vi "SNRvariations.vi"() -> ()   [LabVIEW 2012]
uses:
  <vilib>/addons/Modulation/Digital/General/MT Generate PSK System Parameters(M).vi
  <instrlib>/niUSRP/niUSRP Write Tx Data (CDB Cluster).vi
  <vilib>/addons/Modulation/niDMT.lvlib
panel:
  out "coerced gain":dbl format="%#_6f"
  out "coerced carrier frequency":dbl=100000.0 format="%#_6p"
  in  "IQ rate":dbl=100000.0 format="%#_6p"
  in  "active antenna":string
  in  "Carrier Frequency":dbl
  out "x+y":dbl
  out "Tx Frequency [Hz]":dbl
  out "Enter control signal (1,2 or 3) 2":string
  out "String":string
  in  "millisecond multiple":u32
  out "millisecond timer value":u32
  out "Message Text 2":string
  out "Symbol Rate\n[symbols/sec]":dbl=25000.0 format="%#.6p"
  in  "BPSK System Parameters 9":T1={"Samples per Symbol"=8, "symbol map"=[], "Differential PSK"=enum."disable", "PSK type"=0} caption="BPSK System Parameters" {"PSK type" items=["normal", "shifted", "offset"]; "symbol map" format="%.3f"}
  in  "BPSK System Parameters 8":T1={"Samples per Symbol"=8, "symbol map"=[], "Differential PSK"=enum."disable", "PSK type"=0} caption="BPSK System Parameters" {"PSK type" items=["normal", "shifted", "offset"]; "symbol map" format="%.3f"}
  in  "BPSK System Parameters 7":T1={"Samples per Symbol"=8, "symbol map"=[], "Differential PSK"=enum."disable", "PSK type"=0} caption="BPSK System Parameters" {"PSK type" items=["normal", "shifted", "offset"]; "symbol map" format="%.3f"}
  in  "BPSK System Parameters 6":T1={"Samples per Symbol"=8, "symbol map"=[], "Differential PSK"=enum."disable", "PSK type"=0} caption="BPSK System Parameters" {"PSK type" items=["normal", "shifted", "offset"]; "symbol map" format="%.3f"}
  in  "BPSK System Parameters 5":T1={"Samples per Symbol"=8, "symbol map"=[], "Differential PSK"=enum."disable", "PSK type"=0} caption="BPSK System Parameters" {"PSK type" items=["normal", "shifted", "offset"]; "symbol map" format="%.3f"}
  in  "BPSK System Parameters 4":T1={"Samples per Symbol"=8, "symbol map"=[], "Differential PSK"=enum."disable", "PSK type"=0} caption="BPSK System Parameters" {"PSK type" items=["normal", "shifted", "offset"]; "symbol map" format="%.3f"}
  in  "BPSK System Parameters 3":T1={"Samples per Symbol"=8, "symbol map"=[], "Differential PSK"=enum."disable", "PSK type"=0} caption="BPSK System Parameters" {"PSK type" items=["normal", "shifted", "offset"]; "symbol map" format="%.3f"}
  in  "Tab Control":T2(tab)
  in  "Enter control signal (1,2 or 3)":string
  in  "Packet Parameters":T3={"Guard Bits "=30, "Sync Bits"=20, "Message Bits"=128}
  in  "Packet Pad \n[samples]":i32=200
  in  "Blank Frame \n[samples]":i32=500
  out "Number of Packets in Message":i32=46
  in  "PN sequence order\nfor Sync Bits":i32=31 caption="PN sequence order (9)"
  in  "Packet Repeat":i32=2
  in  "Pulse Shaping Filter Parameters":T4={"Alpha"=0.5, "Filter Length"=6, "TX Filter"=enum."Root Raised Cos"} caption="Pulse Shaping Filter" {"Alpha" format="%.2f"}
  in  "USRP IP address":refnum<k15>="192.168.10.2"
  out "error out":errorcluster
  in  "Queue Length":i32=10
  in  "stop":bool
  out "result":bool
  out "Constellation Graph":T5(graph)
  in  "autoscale":bool
  in  "millisecond multiple 2":u32
  out "millisecond timer value 2":u32
  out "x = y?":bool
  out "Boolean":bool
  out "M-PSK (4)":i32
  # "Guard\nBand"
  # "Sync\nSeq"
  # "Packet\nNumber"
  # "Pad\nData"
  # "Blank\nFrame"
  # "Data"
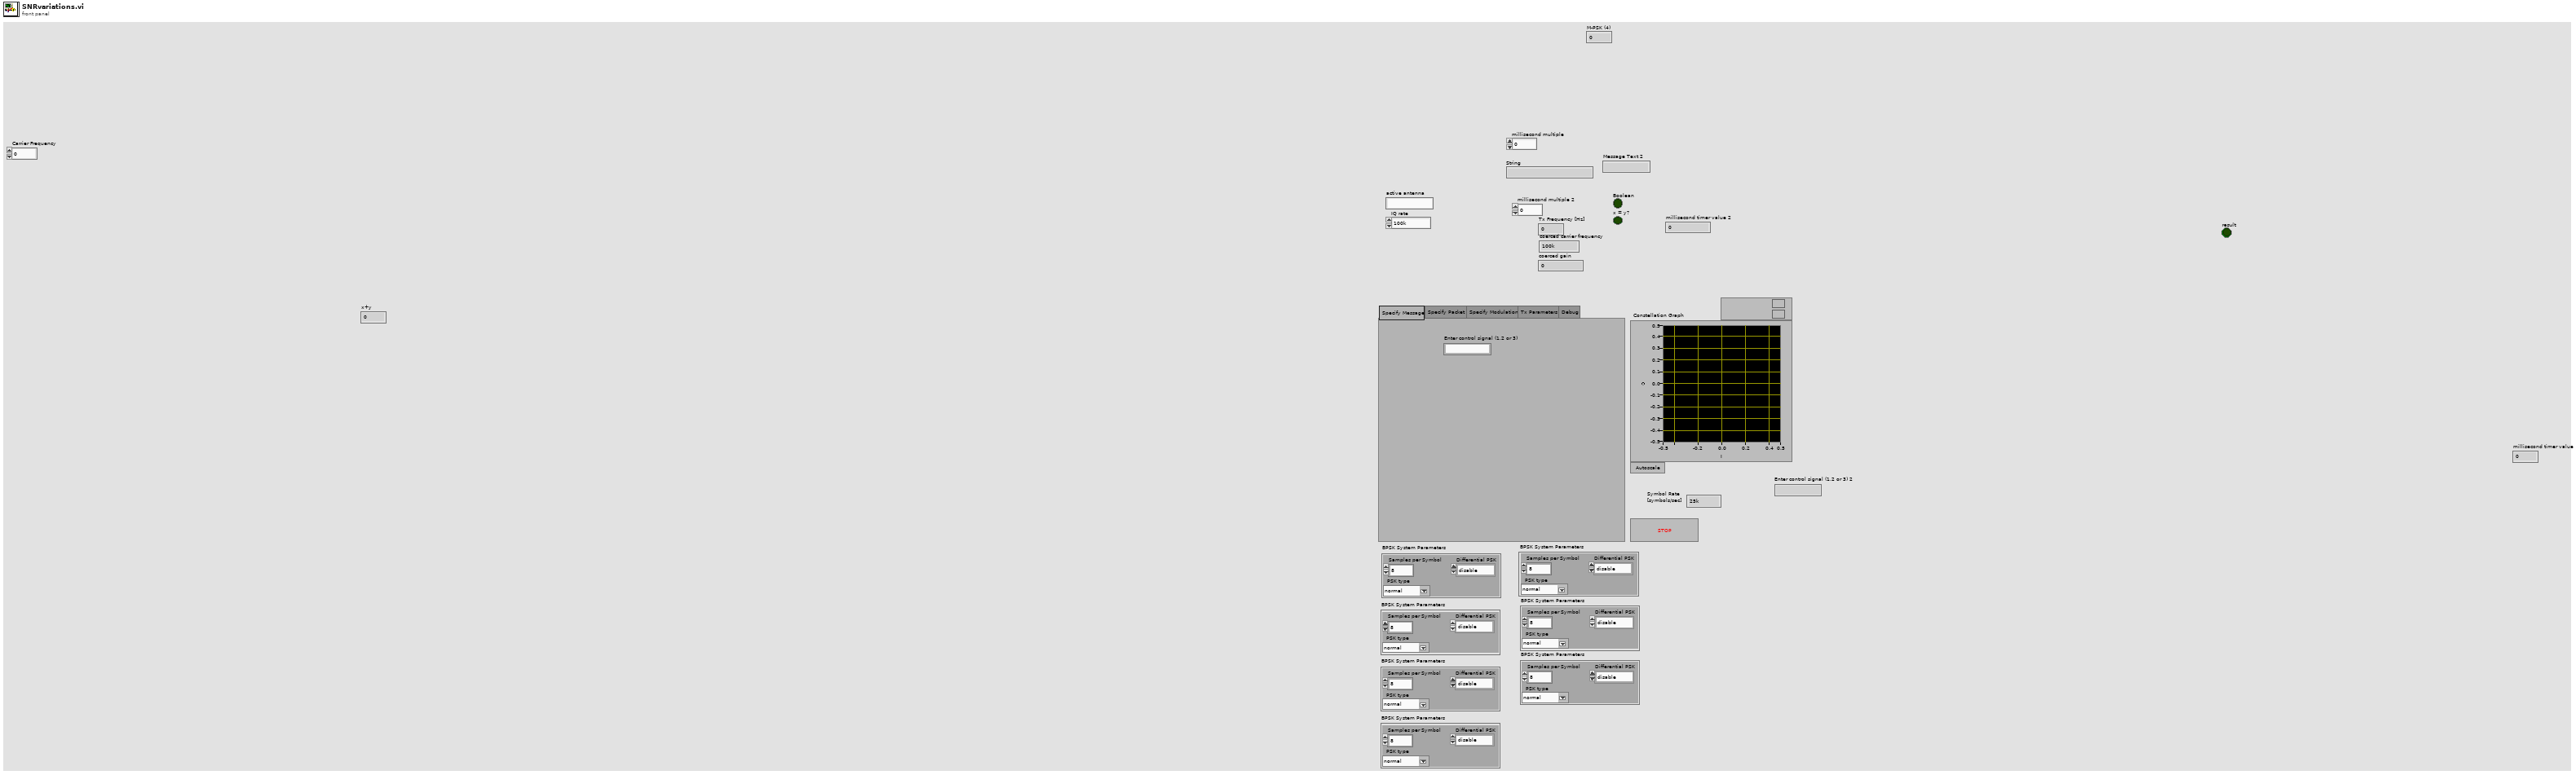
[diagram p1: front panel]
types:
  T1 = cluster{"Samples per Symbol":i32, "symbol map":cdb[], "Differential PSK":enum16{"disable", "enable"}, "PSK type":u16}
  T2 = enum32{"Specify Message", "Specify Packet", "Specify Modulation", "Tx Parameters", "Debug"}
  T3 = cluster{"Guard Bits ":i32, "Sync Bits":i32, "Message Bits":i32}
  T4 = cluster{"Alpha":dbl, "Filter Length":i32, "TX Filter":enum16{"none", "Raised Cosine", "Root Raised Cos", "Gaussian"}}
  T5 = cluster{"Decimated Array":dbl[], "Decimated Array":dbl[]}[]
  T6 = cluster{"samples per symbol (16)":i32, "symbol map":cdb[], "differential PSK":enum16{"disable", "enable"}, "PSK type":u16}
  T7 = cluster{"s? t:f":cluster{"t0":dbl, "dt":dbl, "Y":cdb[]}, i32}
  T8 = cluster{"output complex waveform":cluster{"t0":dbl, "dt":dbl, "Y":cdb[]}, i32}
  T9 = cluster{"constellation":dbl[], "oversampled data":dbl[]}[]
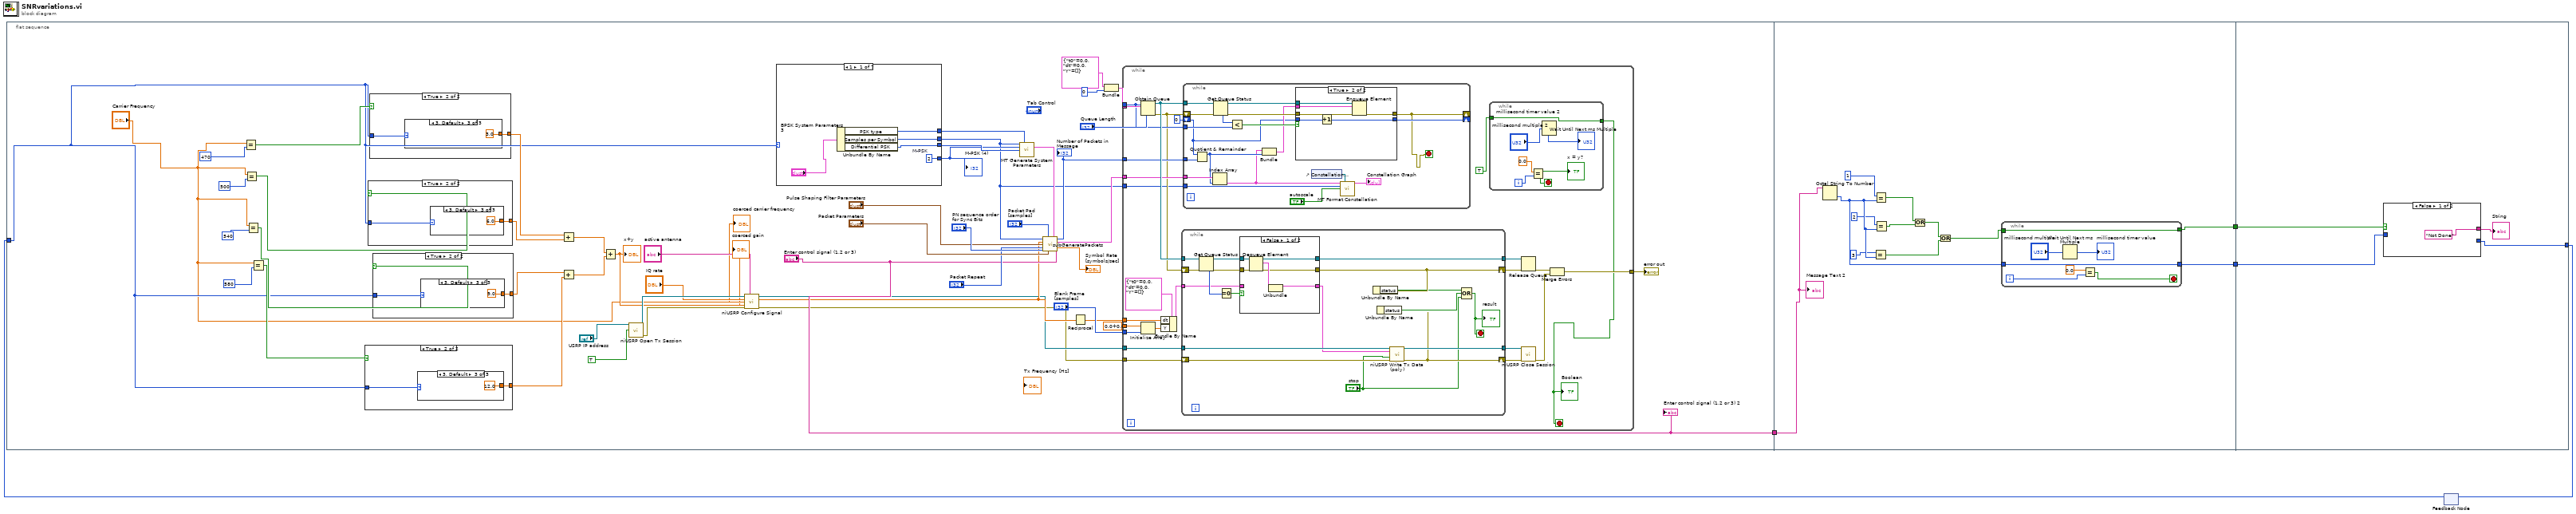
[diagram p0: block diagram]
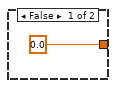
[diagram p2: hidden frame]
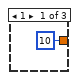
[diagram p3: hidden frame]
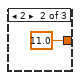
[diagram p4: hidden frame]
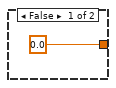
[diagram p5: hidden frame]
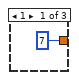
[diagram p6: hidden frame]
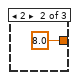
[diagram p7: hidden frame]
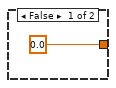
[diagram p8: hidden frame]
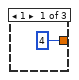
[diagram p9: hidden frame]
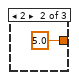
[diagram p10: hidden frame]
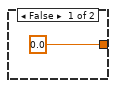
[diagram p11: hidden frame]
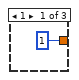
[diagram p12: hidden frame]
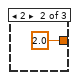
[diagram p13: hidden frame]
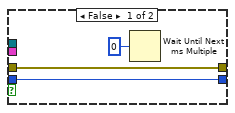
[diagram p14: hidden frame]
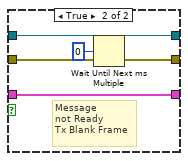
[diagram p15: hidden frame]
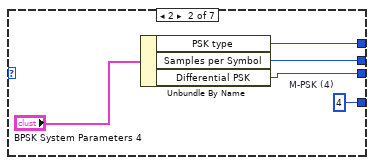
[diagram p16: hidden frame]
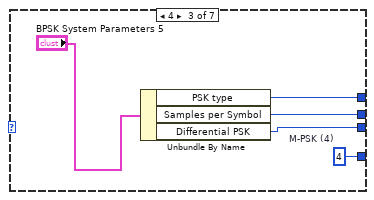
[diagram p17: hidden frame]
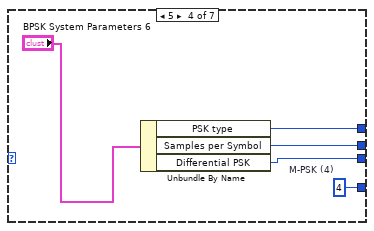
[diagram p18: hidden frame]
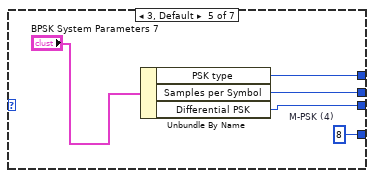
[diagram p19: hidden frame]
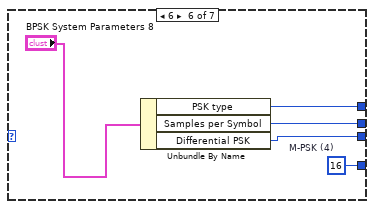
[diagram p20: hidden frame]
diagram:
  n1 = flat-sequence {
    tunnel: ["Enter control signal (1,2 or 3)"] -> w5
    tunnel: w1 -> [w13]
    tunnel: w5 -> [w202]
    tunnel: [w204] -> w4
    tunnel: [w203] -> w3
    tunnel: w4 -> [w223]
    tunnel: w3 -> [w222]
    tunnel: [w221] -> w2
    frame #0 {
      n2 = Equal?(x="Carrier Frequency", y=470) -> (x = y?=w14:bool)
      n3 = Equal?(x="Carrier Frequency", y=500) -> (x = y?=w15:bool)
      n4 = Equal?(x="Carrier Frequency", y=540) -> (x = y?=w16:bool)
      n5 = Equal?(x="Carrier Frequency", y=580) -> (x = y?=w17:bool)
      n6 = case shown="True" w17 {
        tunnel: [0.0 w57] -> w22
        tunnel: w13 -> [_ w58]
        frame False {
        }
        frame True {
          n7 = case shown="3, Default" w58 {
            tunnel: [10 11.0 12.0] -> w57
            frame 1 {
            }
            frame 2 {
            }
            frame 3, Default {
            }
          }
        }
      }
      n8 = case shown="True" w15 {
        tunnel: [0.0 w69] -> w24
        tunnel: w13 -> [_ w70]
        frame False {
        }
        frame True {
          n9 = case shown="3, Default" w70 {
            tunnel: [4 5.0 6.0] -> w69
            frame 1 {
            }
            frame 2 {
            }
            frame 3, Default {
            }
          }
        }
      }
      n10 = case shown="True" w14 {
        tunnel: [0.0 w75] -> w25
        tunnel: w13 -> [_ w76]
        frame False {
        }
        frame True {
          n11 = case shown="3, Default" w76 {
            tunnel: [1 2.0 3.0] -> w75
            frame 1 {
            }
            frame 2 {
            }
            frame 3, Default {
            }
          }
        }
      }
      n12 = case shown="True" w16 {
        tunnel: [0.0 w63] -> w23
        tunnel: w13 -> [_ w64]
        frame False {
        }
        frame True {
          n13 = case shown="3, Default" w64 {
            tunnel: [7 8.0 9.0] -> w63
            frame 1 {
            }
            frame 2 {
            }
            frame 3, Default {
            }
          }
        }
      }
      n14 = Add(x=w25, y=w24) -> (x+y=w27:dbl)
      n15 = Add(x=w23, y=w22) -> (x+y=w26:dbl)
      n16 = Add(x=w27, y=w26) -> (x+y=w12:dbl)
      "x+y" <- w12
      n17 = call <instrlib>:"niUSRP Open Tx Session.vi"("device names"="USRP IP address", "reset"=TRUE) -> ("session handle out"=w30:refnum<k15>, "error out"=w31:errorcluster)  [unwired: 12 in]
      n18 = call <instrlib>:"niUSRP Configure Signal.vi"("session handle"=w30, "IQ rate"="IQ rate", "carrier frequency"="Carrier Frequency", "gain"=w12, "error in (no error)"=w31, "active antenna"="active antenna") -> ("session handle out"=w29:refnum<k15>, "coerced IQ rate"=w32:dbl, "coerced carrier frequency"=→"coerced carrier frequency":dbl, "coerced gain"=→"coerced gain":dbl, "error out"=w28:errorcluster)  [unwired: 5 in]
      n19 = case shown="1" w13 {
        tunnel: [w168 w173 w180 w185 w190 w196 w199] -> w36
        tunnel: [w169 w174 w179 w184 w189 w195 w200] -> w55
        tunnel: [w171 w176 w181 w186 w188 w194 0 ("M-PSK (4)")] -> w47
        tunnel: [w170 w175 w178 w183 w191 w193 w201] -> w41
        frame 1 {
          w171 = 2  # M-PSK
          n20 = Unbundle By Name("BPSK System Parameters 3") -> ("PSK type"=w170:u16, "Samples per Symbol"=w168:i32, "Differential PSK"=w169:enum16{"disable", "enable"})
        }
        frame 2 {
          w176 = 4  # M-PSK (4)
          n21 = Unbundle By Name("BPSK System Parameters 4") -> ("PSK type"=w175:u16, "Samples per Symbol"=w173:i32, "Differential PSK"=w174:enum16{"disable", "enable"})
        }
        frame 4 {
          w181 = 4  # M-PSK (4)
          n22 = Unbundle By Name("BPSK System Parameters 5") -> ("PSK type"=w178:u16, "Samples per Symbol"=w180:i32, "Differential PSK"=w179:enum16{"disable", "enable"})
        }
        frame 5 {
          w186 = 4  # M-PSK (4)
          n23 = Unbundle By Name("BPSK System Parameters 6") -> ("PSK type"=w183:u16, "Samples per Symbol"=w185:i32, "Differential PSK"=w184:enum16{"disable", "enable"})
        }
        frame 3, Default {
          w188 = 8  # M-PSK (4)
          n24 = Unbundle By Name("BPSK System Parameters 7") -> ("PSK type"=w191:u16, "Samples per Symbol"=w190:i32, "Differential PSK"=w189:enum16{"disable", "enable"})
        }
        frame 6 {
          w194 = 16  # M-PSK (4)
          n25 = Unbundle By Name("BPSK System Parameters 8") -> ("PSK type"=w193:u16, "Samples per Symbol"=w196:i32, "Differential PSK"=w195:enum16{"disable", "enable"})
        }
        frame 7 {
          n26 = Unbundle By Name("BPSK System Parameters 9") -> ("PSK type"=w201:u16, "Samples per Symbol"=w199:i32, "Differential PSK"=w200:enum16{"disable", "enable"})
        }
      }
      "M-PSK (4)" <- w47
      n27 = call-poly <vilib>:"MT Generate System Parameters.vi"("samples per symbol (16)"=w36, "PSK type"=w41, "M-PSK (4)"=w47, "differential PSK"=w55) -> ("PSK system parameters"=w42:T6)  [unwired: 9 in, 2 out]
      n28 = call "subGeneratePackets.vi"("Samples per Symbol"=w36, "Packet Pad \n[samples]"="Packet Pad \n[samples]", "PSK system parameters"=w42, "Tx IQ Sampling\nRate [s/sec]"=w32, "Pulse Shaping Filter Parameters"="Pulse Shaping Filter Parameters", "Packet Repeat"="Packet Repeat", "PN sequence order\nfor Sync Bits"="PN sequence order\nfor Sync Bits", "Packet Parameters"="Packet Parameters", "Message Text"="Enter control signal (1,2 or 3)") -> ("Number of Packets"=w46:i32, "Packets"=w49:cluster{"t0":dbl, "dt":dbl, "Y":cdb[]}[], "Symbol Rate"=→"Symbol Rate\n[symbols/sec]":dbl)  [unwired: 4 in]
      "Number of Packets in Message" <- w46
      n29 = Reciprocal(x=w32) -> (1/x=w48:dbl)
      n30 = Bundle("s? t:f"=cluster{"t0":dbl, "dt":dbl, "Y":cdb[]} {"t0"=0.0, "dt"=0.0, "Y"=[]}, 0) -> (w51:T7)  [unwired: 1 in]
      n31 = while {
        tunnel: cdb 0.0+0.0i ("element") -> [w104]
        tunnel: "Blank Frame \n[samples]" -> [w103]
        tunnel: w51 -> [w97]
        tunnel: "Queue Length" -> [w95]
        tunnel: w49 -> [w94]
        tunnel: w28 -> [w93]
        tunnel: w48 -> [w90]
        tunnel: w29 -> [w89]
        tunnel: w46 -> [w88]
        tunnel: [w83] -> w40
        tunnel: w36 -> [w82]
        stop <- w80 stop-if-true
        n32 = Obtain Queue(max queue size (-1, unlimited)=w95, element data type=w97) -> (queue out=w102:refnum<queue>, error out=w86:errorcluster)  [unwired: 3 in, 1 out]
        n33 = Initialize Array(w104, w103) -> (w101:cdb[])
        n34 = Bundle By Name(cluster=cluster{"t0":dbl, "dt":dbl, "Y":cdb[]} {"t0"=0.0, "dt"=0.0, "Y"=[]} ("s? t:f"), "dt"=w90, "Y"=w101) -> (w100:cluster{"t0":dbl, "dt":dbl, "Y":cdb[]})
        n35 = while {
          tunnel: w89 -> [w147]
          shift-right: [w144] -> w92
          shift-left: w93 -> [w148]
          tunnel: w102 -> [w156]
          tunnel: w100 -> [w153]
          tunnel: [w152] -> w99
          tunnel: [w146] -> w91
          shift-right: [w142] -> w98
          shift-left: w86 -> [w149]
          stop <- w139 stop-if-true
          n36 = Get Queue Status(queue=w156, error in (no error)=w149) -> (queue out=w151:refnum<queue>, error out=w150:errorcluster, # elements in queue=w155:i32)  [unwired: 1 in, 5 out]
          n37 = Equal To 0?(x=w155) -> (x = 0?=w154:bool)
          n38 = case shown="False" w154 {
            tunnel: w153 -> [_ w166]
            tunnel: [w158 w166] -> w140
            tunnel: [w162 w164] -> w152
            tunnel: [w157 w165] -> w142
            tunnel: w151 -> [w161 w164]
            tunnel: w150 -> [w160 w165]
            frame False {
              n39 = Dequeue Element(queue=w161, error in (no error)=w160) -> (queue out=w162:refnum<queue>, element=w159:T7, error out=w157:errorcluster)  [unwired: 1 in, 1 out]
              n40 = Unbundle(w159) -> ("s? t:f"=w158:cluster{"t0":dbl, "dt":dbl, "Y":cdb[]})  [unwired: 1 out]
            }
            frame True {
              # "Message\nnot Ready\nTx Blank Frame"
              n41 = Wait Until Next ms Multiple(millisecond multiple=u32 0) -> ()  [unwired: 1 out]
            }
          }
          n42 = Unbundle By Name(w142) -> ("status"=w141:bool)
          n43 = call-poly <instrlib>:"niUSRP Write Tx Data (poly).vi"("session handle"=w147, "data"=w140, "end of data?"="stop", "error in (no error)"=w148) -> ("session handle out"=w146:refnum<k15>, "error out"=w144:errorcluster)  [unwired: 10 in]
          n44 = Unbundle By Name(w144) -> ("status"=w145:bool)
          n45 = Compound Arithmetic op=OR(w141, w145, "stop") -> (w139:bool)
          "result" <- w139
        }
        n46 = while {
          tunnel: w102 -> [w129]
          shift-right: [w122] -> _
          shift-left: 0 -> [w118]
          tunnel: w94 -> [w119]
          tunnel: w95 -> [w121]
          tunnel: w88 -> [w120]
          shift-right: [w111] -> _
          shift-left: w86 -> [w124]
          tunnel: w82 -> [w114]
          stop <- w111 stop-if-true
          n47 = Quotient & Remainder(x=w118, y=w120) -> (x-y*floor(x/y)=w117:i32)  [unwired: 1 out]
          n48 = Index Array(array=w119, index=w117) -> (element=w112:cluster{"t0":dbl, "dt":dbl, "Y":cdb[]})
          n49 = Get Queue Status(queue=w129, error in (no error)=w124) -> (queue out=w128:refnum<queue>, error out=w125:errorcluster, # elements in queue=w127:i32)  [unwired: 1 in, 5 out]
          n50 = Less?(x=w127, y=w121) -> (x < y?=w126:bool)
          n51 = Bundle("output complex waveform"=w112, w117) -> (w123:T8)  [unwired: 1 in]
          n52 = case shown="True" w126 {
            tunnel: w125 -> [w130 w138]
            tunnel: w128 -> [_ w137]
            tunnel: [w130 w136] -> w111
            tunnel: w123 -> [_ w135]
            tunnel: w118 -> [w132 w134]
            tunnel: [w132 w133] -> w122
            frame False {
              n53 = Wait Until Next ms Multiple(millisecond multiple=u32 0) -> ()  [unwired: 1 out]
            }
            frame True {
              n54 = Increment(x=w134) -> (x+1=w133:i32)
              n55 = Enqueue Element(queue=w137, element=w135, error in (no error)=w138) -> (error out=w136:errorcluster)  [unwired: 1 in, 2 out]
            }
          }
          n56 = control-ref of="Constellation Graph"() -> (w115:refnum<vi>)
          n57 = call <vilib>:"MT Format Constellation.vi"("waveform"=w112, "constellation reference"=w115, "samples per symbol"=w114, "autoscale"="autoscale") -> ("constellation graph"=→"Constellation Graph":T9)  [unwired: 1 in, 10 out]
        }
        n58 = while {
          tunnel: TRUE -> [w110]
          tunnel: [w110] -> w80
          i -> [w108]
          stop <- w107 stop-if-true
          n59 = Equal?(x=0.0, y=w108) -> (x = y?=w107:bool)
          "x = y?" <- w107
          n60 = Wait Until Next ms Multiple(millisecond multiple="millisecond multiple 2") -> (millisecond timer value=→"millisecond timer value 2":u32)
        }
        "Boolean" <- w80
        n61 = Release Queue(queue=w99, error in (no error)=w98) -> (error out=w85:errorcluster)  [unwired: 3 out]
        n62 = call <instrlib>:"niUSRP Close Session.vi"("session handle"=w91, "error in (no error)"=w92) -> ("error out"=w84:errorcluster)  [unwired: 13 in]
        n63 = Merge Errors(w85, w84) -> (w83:errorcluster)
      }
      "error out" <- w40
      "Enter control signal (1,2 or 3) 2" <- "Enter control signal (1,2 or 3)"
    }
    frame #1 {
      n64 = Octal String To Number(4:w202) -> (0:w208:u32)  [unwired: 2 in, 1 out]
      n65 = Equal?(x=3, y=w208) -> (x = y?=w210:bool)
      n66 = Equal?(x=1, y=w208) -> (x = y?=w213:bool)
      n67 = Equal?(x=2, y=w208) -> (x = y?=w212:bool)
      n68 = Or(x=w213, y=w212) -> (x .or. y?=w211:bool)
      n69 = Or(x=w211, y=w210) -> (x .or. y?=w209:bool)
      n70 = while {
        tunnel: w209 -> [w218]
        tunnel: [w218] -> w204
        tunnel: w208 -> [w217]
        tunnel: [w217] -> w203
        i -> [w215]
        stop <- w214 stop-if-true
        n71 = Wait Until Next ms Multiple(millisecond multiple="millisecond multiple") -> (millisecond timer value=→"millisecond timer value":u32)
        n72 = Equal?(x=0.0, y=w215) -> (x = y?=w214:bool)
      }
      "Message Text 2" <- w202
    }
    frame #2 {
      n73 = case shown="False" w223 {
        tunnel: ["Not Done" "Switching Done"] -> w224
        tunnel: [_ w226] -> w221
        tunnel: w222 -> [_ w226]
        frame False {
        }
        frame True {
        }
      }
      "String" <- w224
    }
  }
  n74 = feedback #1() -> (w1:u32)  [unwired: 1 in]
  n75 = feedback-in #1(w2) -> ()
